vi "G_3d2.vi"() -> ()   [LabVIEW 2012]
panel:
  out "obs":refnum<vi>
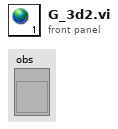
[diagram p1: front panel]
diagram:
